vi "Band.vi"   [LabVIEW 2017, in "VibrationAnalysisFunctions.lvlib"]
uses:
  <vilib>/addons/InsightCM/Utilities/Analysis/Vibration/VibrationAnalysisFunctions.lvlib
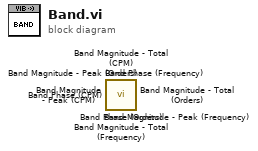
[diagram p0: block diagram]
diagram:
  n1 = call <vilib>:"Band Phase (Orders).vi"() -> ()  [unwired: 14 in, 2 out]
  n2 = call <vilib>:"Band Phase (Frequency).vi"() -> ()  [unwired: 14 in, 2 out]
  n3 = call <vilib>:"Band Phase (CPM).vi"() -> ()  [unwired: 14 in, 2 out]
  n4 = call <vilib>:"Band Magnitude - Total (Orders).vi"() -> ()  [unwired: 14 in, 2 out]
  n5 = call <vilib>:"Band Magnitude - Total (Frequency).vi"() -> ()  [unwired: 14 in, 2 out]
  n6 = call <vilib>:"Band Magnitude - Total (CPM).vi"() -> ()  [unwired: 14 in, 2 out]
  n7 = call <vilib>:"Band Magnitude - Peak (Orders).vi"() -> ()  [unwired: 14 in, 2 out]
  n8 = call <vilib>:"Band Magnitude - Peak (Frequency).vi"() -> ()  [unwired: 14 in, 2 out]
  n9 = call <vilib>:"Band Magnitude - Peak (CPM).vi"() -> ()  [unwired: 14 in, 2 out]
